vi "String Value to dot Net.vi"(7 "image path":path, 8 "error in (no error)":errorcluster, 10 "element":string, 11 "GridColumn in":refnum<class "GridColumn.lvclass">) -> (0 "error out":errorcluster, 3 ".NET object":refnum<k24>)   [LabVIEW 2013, in "DataGrid.lvlib" / "DataTable.lvclass"]
uses:
  DataTable.lvclass
  GridColumn/GridColumn.lvclass
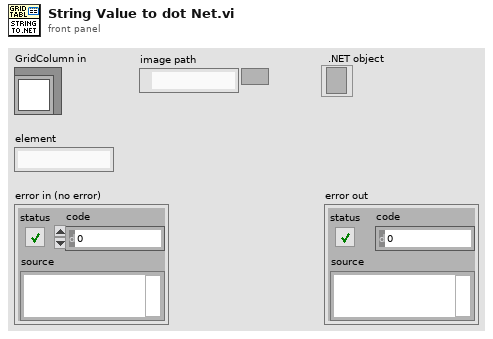
[diagram p1: front panel]
types:
  T1 = typedef "DataGrid.lvlib/GridColumn.lvclass/ColumnType.ctl" = enum16{"string", "image", "check", "numeric", "timestamp", "button", "combo", "link"}
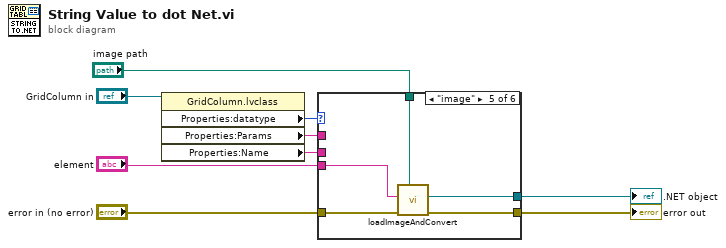
[diagram p0: block diagram]
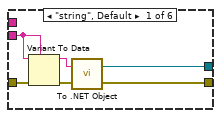
[diagram p2: hidden frame]
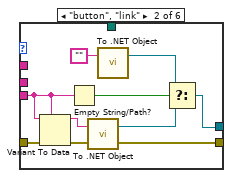
[diagram p3: hidden frame]
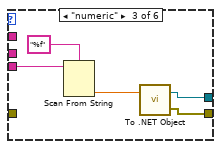
[diagram p4: hidden frame]
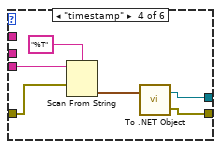
[diagram p5: hidden frame]
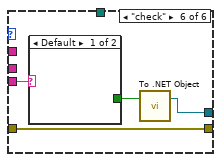
[diagram p6: hidden frame]
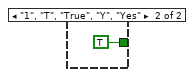
[diagram p7: hidden frame]
diagram:
  n1 = property class="GridColumn.lvclass"(reference="GridColumn in") -> ("Properties:datatype"=w9:T1, "Properties:Params"=w8:string, "Properties:Name"=w7:string)  [unwired: 1 in, 2 out]
  n2 = case shown="\"image\"" w9 {
    tunnel: "element" -> [w11 w21 w28 w34 w41 w43]
    tunnel: [w10 w18 w29 w35 w40 w44] -> w3
    tunnel: "error in (no error)" -> [w14 w24 _ w32 w39 w45]
    tunnel: [w12 w22 w30 w36 w38 w45] -> w2
    tunnel: w8 -> [_ _ _ _ _ _]
    tunnel: w7 -> [_ _ _ _ _ _]
    tunnel: "image path" -> [_ _ _ _ w37 _]
    frame "string", Default {
      n3 = Variant To Data(error in=w14, type=w11, Variant=w11) -> (data=w15:string, error out=w13:errorcluster)
      n4 = call <vilib>:"To .NET Object.vi"("error in (no error)"=w13, "anything"=w15) -> ("error out"=w12:errorcluster, ".NET object"=w10:refnum<k24>)
    }
    frame "button", "link" {
      n5 = Variant To Data(error in=w24, type=w21, Variant=w21) -> (data=w25:string, error out=w23:errorcluster)
      n6 = Empty String/Path?(string/path=w21) -> (empty?=w20:bool)
      n7 = call <vilib>:"To .NET Object.vi"("error in (no error)"=w23, "anything"=w25) -> ("error out"=w22:errorcluster, ".NET object"=w19:refnum<k24>)
      n8 = call <vilib>:"To .NET Object.vi"("anything"="") -> (".NET object"=w16:refnum<k24>)  [unwired: 1 in, 1 out]
      n9 = Select(t=w16, s=w20, f=w19) -> (s? t:f=w18:refnum<k24>)
    }
    frame "numeric" {
      n10 = Scan From String(format string="%f", input string=w28) -> (output 1=w26:dbl)  [unwired: 3 in, 3 out]
      n11 = call <vilib>:"To .NET Object.vi"("anything"=w26) -> ("error out"=w30:errorcluster, ".NET object"=w29:refnum<k24>)  [unwired: 1 in]
    }
    frame "timestamp" {
      n12 = Scan From String(format string="%T", input string=w34, error in=w32) -> (output 1=w31:timestamp)  [unwired: 2 in, 3 out]
      n13 = call <vilib>:"To .NET Object.vi"("anything"=w31) -> ("error out"=w36:errorcluster, ".NET object"=w35:refnum<k24>)  [unwired: 1 in]
    }
    frame "image" {
      n14 = call "loadImageAndConvert.vi"("image path"=w37, "error in (no error)"=w39, "name or relative path"=w41) -> ("error out"=w38:errorcluster, ".NET object"=w40:refnum<k24>)  [unwired: 7 in]
    }
    frame "check" {
      n15 = case shown="Default" w43 {
        tunnel: [_ TRUE] -> w42
        frame Default {
        }
        frame "1", "T", "True", "Y", "Yes" {
        }
      }
      n16 = call <vilib>:"To .NET Object.vi"("anything"=w42) -> (".NET object"=w44:refnum<k24>)  [unwired: 1 in, 1 out]
    }
  }
  "error out" <- w2
  ".NET object" <- w3
